vi "testFlattenVelocityToXML.vi"() -> ()   [LabVIEW 2012, in "UnitsAndXML.lvlib"]
uses:
  <userlib>/Common/UnitsAndXML/UnitsAndXML.lvlib
  <userlib>/Common/UnitsAndXML/FlattenItemWithUnitToXML/FlattenVelocityToXML/VelocityUnit.ctl
  <userlib>/Common/UnitsAndXML/FlattenItemWithUnitToXML/FlattenVelocityToXML/typeMethods/flattenVelocityToXML_Array.vi
  <userlib>/Common/UnitsAndXML/FlattenItemWithUnitToXML/FlattenVelocityToXML/typeMethods/flattenVelocityToXML_Scalar.vi
panel:
  out "error out":errorcluster
  in  "velocityUnitInXML":T1
  out "xmlStringArray":string
  out "xmlStringScalar":string
  in  "velocity":dbl[unit][](array[numeric])=[7.716666666666666, 15.433333333333332, 23.150000000000002, 30.866666666666664]
  in  "velocity":dbl[unit]=7.716666666666667
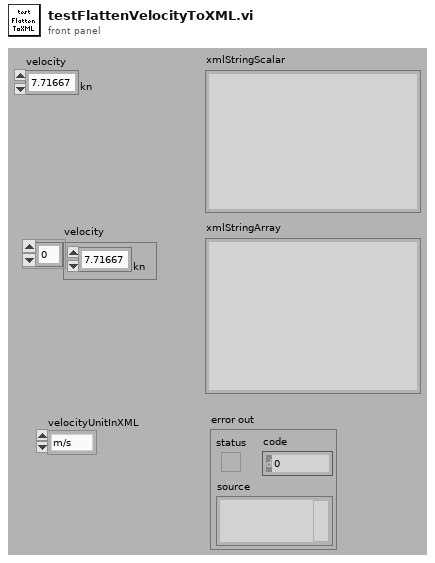
[diagram p1: front panel]
types:
  T1 = typedef "UnitsAndXML.lvlib/VelocityUnit.ctl" = enum16{"m/s", "km/s", "kn"}
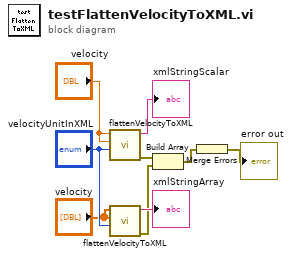
[diagram p0: block diagram]
diagram:
  n1 = call-poly <userlib>:"flattenVelocityToXML.vi"("velocityUnitInXML"="velocityUnitInXML", "velocityAgain"="velocity", "velocity"="velocity") -> ("error out"=w6:errorcluster, "xmlString"=→"xmlStringScalar":string)  [unwired: 7 in]
  n2 = call-poly <userlib>:"flattenVelocityToXML.vi"("velocityUnitInXML"="velocityUnitInXML", "velocityAgain"="velocity", "velocity"="velocity") -> ("error out"=w1:errorcluster, "xmlString"=→"xmlStringArray":string)  [unwired: 7 in]
  n3 = Build Array(w6, w1) -> (w7:errorcluster[])
  n4 = Merge Errors(w7) -> (→"error out":errorcluster)
